vi "mobility_subvi_07_12a_JW.vi"(9 "NumPts":dbl=5.0, 11 "Path":path) -> (0 "Index-Lin":dbl, 1 "Index-Sat":dbl, 2 "Output":T1, 3 "XY Graph-Sat":cluster{dbl[], dbl[]}[](graph))   [LabVIEW 2011]
uses:
  <vilib>/Utility/file.llb/Read From Spreadsheet File (string).vi
  <vilib>/Analysis/NI_AALPro.lvlib
panel:
  out "XY Graph-Lin":cluster{dbl[], dbl[]}[](graph)
  out "ID Column 2":string[][](table)
  out "Capacitance (C)":dbl
  out "Numeric":dbl
  out "Dielectric (nm)":string
  out "Dielectric (d)":dbl
  out "Width":dbl
  out "Length":dbl
  out "ID Column 3":string[][](table)
  out "Vg Column":string[][](table)
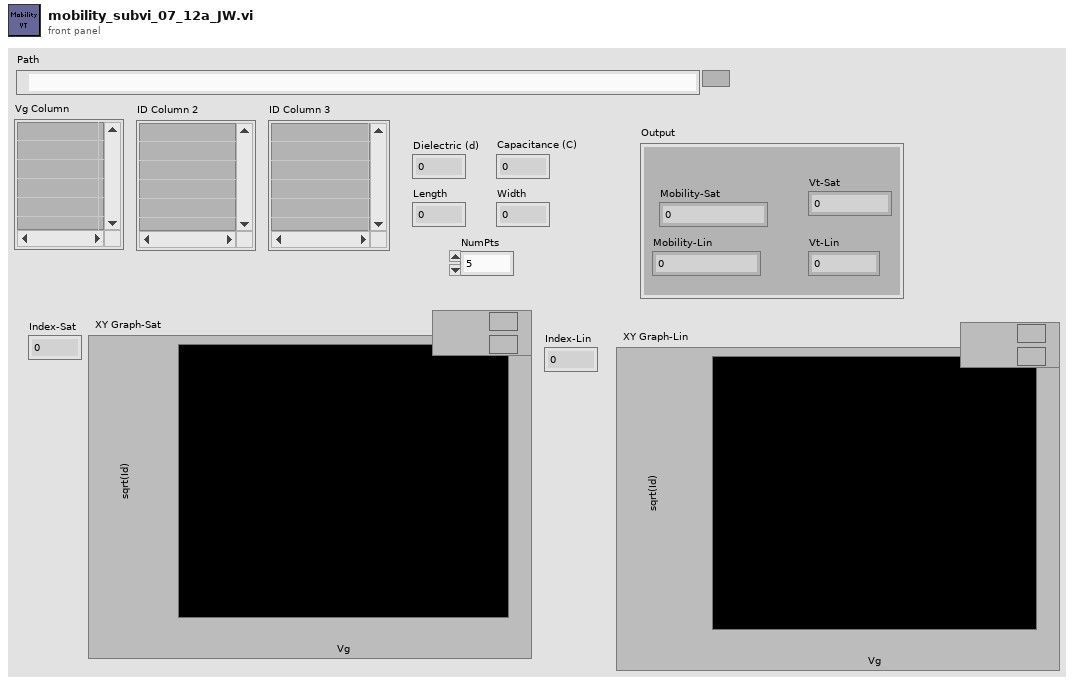
[diagram p1: front panel]
types:
  T1 = cluster{"Mobility-Sat":dbl, "Vt-Sat":dbl, "Vt-Lin":dbl, "Mobility-Lin":dbl}
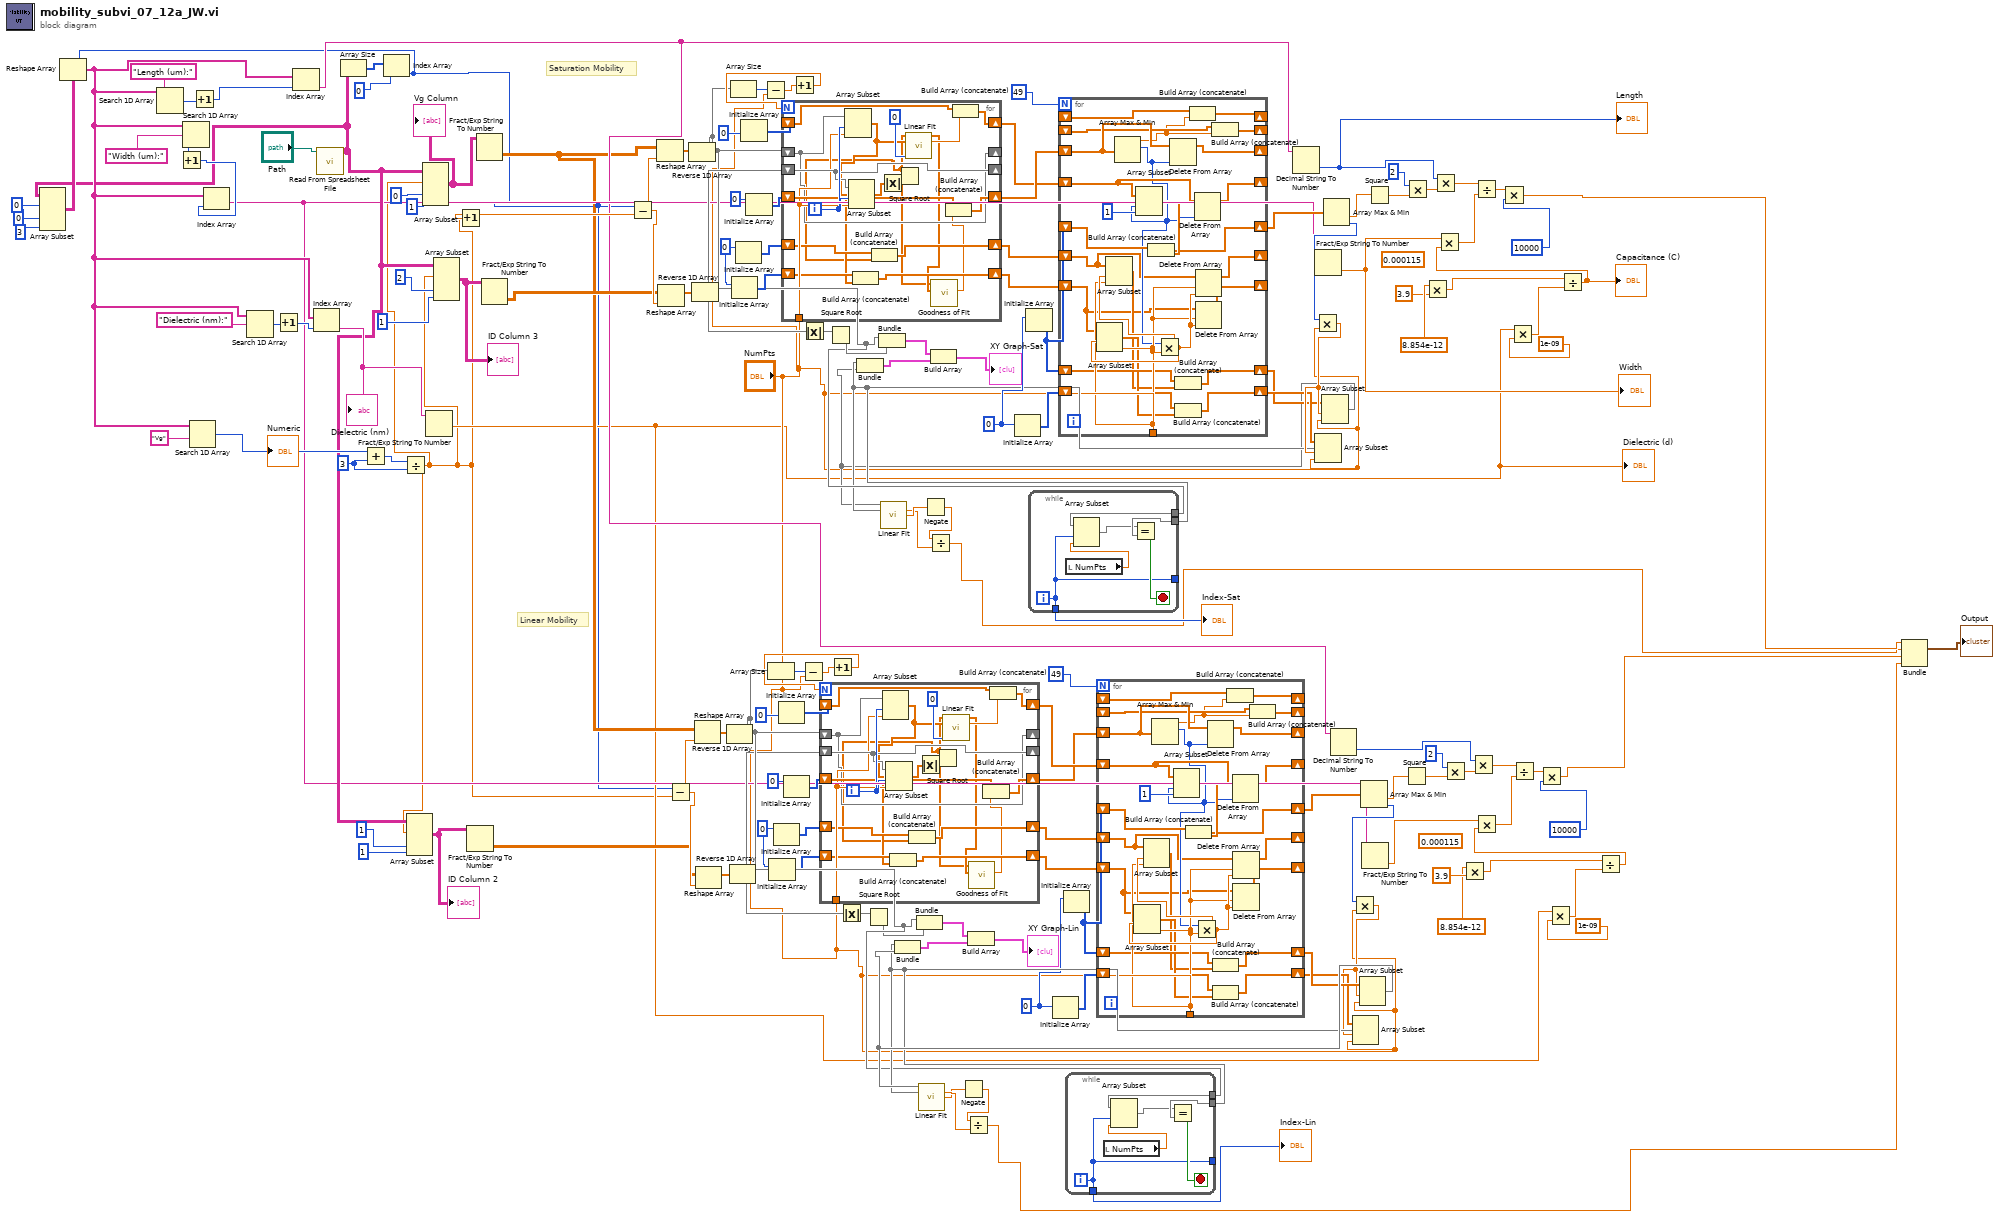
[diagram p0: block diagram]
diagram:
  w24 = 0
  w33 = 0
  (unwired) 0.000115
  w75 = 3
  w146 = 0
  w137 = 0
  (unwired) 0.000115
  # "Linear Mobility"
  # "Saturation Mobility"
  n1 = call-poly <vilib>:"Read From Spreadsheet File.vi"("file path (dialog if empty)"="Path") -> ("all rows"=w72:string[][])  [unwired: 6 in, 4 out]
  n2 = Array Subset(array=w72, index (row)=0, index (col)=0, length (col)=3) -> (w122:string[][])  [unwired: 1 in]
  n3 = Array Size(array=w72) -> (size(s)=w127:i32[])
  n4 = Index Array(array=w127, index=0) -> (element=w6:i32)
  n5 = Reshape Array(w122, w6) -> (w74:string[])
  n6 = Search 1D Array(1D array=w74, element="Length (um):") -> (index of element=w115:i32)  [unwired: 1 in]
  n7 = Search 1D Array(1D array=w74, element="Width (um):") -> (index of element=w116:i32)  [unwired: 1 in]
  n8 = Increment(x=w116) -> (x+1=w120:i32)
  n9 = Search 1D Array(1D array=w74, element="Vg") -> (index of element=w77:i32)  [unwired: 1 in]
  "Numeric" <- w77
  n10 = Increment(x=w115) -> (x+1=w118:i32)
  n11 = Index Array(array=w74, index=w120) -> (element=w13:string)
  n12 = Search 1D Array(1D array=w74, element="Dielectric (nm):") -> (index of element=w86:i32)  [unwired: 1 in]
  n13 = Increment(x=w86) -> (x+1=w85:i32)
  n14 = Index Array(array=w74, index=w118) -> (element=w12:string)
  n15 = Index Array(array=w74, index=w85) -> (element=w84:string)
  "Dielectric (nm)" <- w84
  n16 = Add(x=w77, y=w75) -> (x+y=w76:i32)
  n17 = Divide(x=w76, y=w75) -> (x/y=w7:dbl)
  n18 = Array Subset(array=w72, index (row)=w7, index (col)=1, length (col)=1) -> (w69:string[][])  [unwired: 1 in]
  "ID Column 2" <- w69
  n19 = Array Subset(array=w72, index (row)=w7, index (col)=0, length (col)=1) -> (w108:string[][])  [unwired: 1 in]
  "Vg Column" <- w108
  n20 = Fract/Exp String To Number(string=w84) -> (number=w8:dbl)  [unwired: 3 in, 1 out]
  "Dielectric (d)" <- w8
  n21 = Array Subset(array=w72, index (row)=w7, index (col)=2, length (col)=1) -> (w109:string[][])  [unwired: 1 in]
  "ID Column 3" <- w109
  n22 = Increment(x=w7) -> (x+1=w154:dbl)
  n23 = Fract/Exp String To Number(string=w69) -> (number=w9:dbl[][])  [unwired: 3 in, 1 out]
  n24 = Fract/Exp String To Number(string=w108) -> (number=w10:dbl[][])  [unwired: 3 in, 1 out]
  n25 = Fract/Exp String To Number(string=w109) -> (number=w110:dbl[][])  [unwired: 3 in, 1 out]
  n26 = Subtract(x=w6, y=w154) -> (x-y=w155:dbl)
  n27 = Reshape Array(w10, w155) -> (w142:dbl[])
  n28 = Reshape Array(w110, w155) -> (w143:dbl[])
  n29 = Subtract(x=w6, y=w7) -> (x-y=w16:dbl)
  n30 = Reverse 1D Array(array=w142) -> (reversed array=w89:dbl[])
  n31 = Reverse 1D Array(array=w143) -> (reversed array=w144:dbl[])
  n32 = Reshape Array(w10, w16) -> (w28:dbl[])
  n33 = Reshape Array(w9, w16) -> (w27:dbl[])
  n34 = Reverse 1D Array(array=w28) -> (reversed array=w61:dbl[])
  n35 = Reverse 1D Array(array=w27) -> (reversed array=w26:dbl[])
  n36 = Array Size(array=w89) -> (size(s)=w102:i32)
  n37 = Initialize Array(w137) -> (w139:i32[])  [unwired: 1 in]
  n38 = Initialize Array(w137) -> (w138:i32[])  [unwired: 1 in]
  n39 = Initialize Array(0) -> (w103:i32[])  [unwired: 1 in]
  n40 = Initialize Array(0) -> (w104:i32[])  [unwired: 1 in]
  n41 = Subtract(x=w102, y="NumPts") -> (x-y=w156:dbl)
  n42 = Array Size(array=w61) -> (size(s)=w53:i32)
  n43 = Initialize Array(w33) -> (w31:i32[])  [unwired: 1 in]
  n44 = Initialize Array(w33) -> (w32:i32[])  [unwired: 1 in]
  n45 = Initialize Array(0) -> (w52:i32[])  [unwired: 1 in]
  n46 = Initialize Array(0) -> (w51:i32[])  [unwired: 1 in]
  n47 = Increment(x=w156) -> (x+1=w157:dbl)
  n48 = for {
    N: w157 -> [_]
    shift-right: [w162] -> _
    shift-left: w89 -> [w162]
    shift-right: [w171] -> _
    shift-left: w144 -> [w171]
    shift-right: [w175] -> w112
    shift-left: w103 -> [w174]
    shift-right: [w173] -> w128
    shift-left: w104 -> [w172]
    tunnel: "NumPts" -> [w167]
    shift-right: [w165] -> w140
    shift-left: w138 -> [w166]
    shift-right: [w163] -> w141
    shift-left: w139 -> [w164]
    i -> [w177]
    n49 = Array Subset(array=w162, index=w177, length=w167) -> (w161:dbl[])
    n50 = Array Subset(array=w171, index=w177, length=w167) -> (w170:dbl[])
    n51 = Build Array (concatenate)(w164, w161) -> (w163:dbl[])
    n52 = Absolute Value(x=w170) -> (abs(x)=w169:dbl[])
    n53 = Square Root(x=w169) -> (sqrt(x)=w158:dbl[])
    n54 = Build Array (concatenate)(w166, w158) -> (w165:dbl[])
    n55 = call <vilib>:"Linear Fit.vi"("Y"=w158, "X"=w161, "method"=0) -> ("Best Linear Fit"=w160:dbl[], "slope"=w176:dbl)  [unwired: 8 in, 3 out]
    n56 = call <vilib>:"Goodness of Fit.vi"("Best Fit"=w160, "Y"=w158) -> ("R-square"=w159:dbl)  [unwired: 6 in, 3 out]
    n57 = Build Array (concatenate)(w172, w159) -> (w173:dbl[])
    n58 = Build Array (concatenate)(w174, w176) -> (w175:dbl[])
  }
  n59 = Subtract(x=w53, y="NumPts") -> (x-y=w15:dbl)
  n60 = Absolute Value(x=w144) -> (abs(x)=w136:dbl[])
  n61 = Square Root(x=w136) -> (sqrt(x)=w153:dbl[])
  n62 = Increment(x=w15) -> (x+1=w14:dbl)
  n63 = for {
    N: w14 -> [_]
    shift-right: [w182] -> _
    shift-left: w61 -> [w182]
    shift-right: [w191] -> _
    shift-left: w26 -> [w191]
    shift-right: [w195] -> w46
    shift-left: w52 -> [w194]
    shift-right: [w193] -> w42
    shift-left: w51 -> [w192]
    tunnel: "NumPts" -> [w187]
    shift-right: [w185] -> w30
    shift-left: w32 -> [w186]
    shift-right: [w183] -> w29
    shift-left: w31 -> [w184]
    i -> [w197]
    n64 = Array Subset(array=w182, index=w197, length=w187) -> (w181:dbl[])
    n65 = Array Subset(array=w191, index=w197, length=w187) -> (w190:dbl[])
    n66 = Build Array (concatenate)(w184, w181) -> (w183:dbl[])
    n67 = Absolute Value(x=w190) -> (abs(x)=w189:dbl[])
    n68 = Square Root(x=w189) -> (sqrt(x)=w178:dbl[])
    n69 = Build Array (concatenate)(w186, w178) -> (w185:dbl[])
    n70 = call <vilib>:"Linear Fit.vi"("Y"=w178, "X"=w181, "method"=0) -> ("Best Linear Fit"=w180:dbl[], "slope"=w196:dbl)  [unwired: 8 in, 3 out]
    n71 = call <vilib>:"Goodness of Fit.vi"("Best Fit"=w180, "Y"=w178) -> ("R-square"=w179:dbl)  [unwired: 6 in, 3 out]
    n72 = Build Array (concatenate)(w192, w179) -> (w193:dbl[])
    n73 = Build Array (concatenate)(w194, w196) -> (w195:dbl[])
  }
  n74 = Absolute Value(x=w26) -> (abs(x)=w34:dbl[])
  n75 = Square Root(x=w34) -> (sqrt(x)=w17:dbl[])
  n76 = Bundle(w89, w153) -> (w135:cluster{dbl[], dbl[]})  [unwired: 1 in]
  n77 = Bundle(w61, w17) -> (w35:cluster{dbl[], dbl[]})  [unwired: 1 in]
  n78 = Initialize Array(w146) -> (w145:i32[])  [unwired: 1 in]
  n79 = Initialize Array(w146) -> (w150:i32[])  [unwired: 1 in]
  n80 = Initialize Array(w24) -> (w25:i32[])  [unwired: 1 in]
  n81 = for {
    N: 49 -> [_]
    shift-right: [w222] -> _
    shift-left: w128 -> [w223]
    shift-right: [w202] -> _
    shift-left: w112 -> [w203]
    shift-right: [w219] -> w117
    shift-left: w150 -> [w218]
    shift-right: [w217] -> _
    shift-left: _ -> [w216]
    shift-right: [w215] -> _
    shift-left: _ -> [w214]
    shift-right: [w213] -> _
    shift-left: w140 -> [w199]
    shift-right: [w211] -> _
    shift-left: w141 -> [w198]
    tunnel: "NumPts" -> [w210]
    shift-right: [w209] -> w147
    shift-left: w150 -> [w208]
    shift-right: [w207] -> w148
    shift-left: w145 -> [w206]
    n82 = Array Max & Min(array=w223) -> (max value=w201:dbl, max index (indices)=w200:i32)  [unwired: 2 out]
    n83 = Array Subset(array=w203, index=w200, length=1) -> (w220:dbl[])
    n84 = Build Array (concatenate)(w218, w220) -> (w219:dbl[])
    n85 = Multiply(x=w200, y=w210) -> (x*y=w212:dbl)
    n86 = Array Subset(array=w198, index=w212, length=w210) -> (w205:dbl[])
    n87 = Array Subset(array=w199, index=w212, length=w210) -> (w204:dbl[])
    n88 = Delete From Array(array=w223, index=w200) -> (array with subset deleted=w222:dbl[])  [unwired: 1 in, 1 out]
    n89 = Build Array (concatenate)(w208, w204) -> (w209:dbl[])
    n90 = Build Array (concatenate)(w206, w205) -> (w207:dbl[])
    n91 = Build Array (concatenate)(w216, w201) -> (w217:dbl[])
    n92 = Delete From Array(array=w203, index=w200) -> (array with subset deleted=w202:dbl[])  [unwired: 1 in, 1 out]
    n93 = Delete From Array(array=w199, length=w210, index=w212) -> (array with subset deleted=w213:dbl[])  [unwired: 1 out]
    n94 = Delete From Array(array=w198, length=w210, index=w212) -> (array with subset deleted=w211:dbl[])  [unwired: 1 out]
    n95 = Build Array (concatenate)(w214, w201) -> (w215:dbl[])
  }
  n96 = Initialize Array(w24) -> (w20:i32[])  [unwired: 1 in]
  n97 = for {
    N: 49 -> [_]
    shift-right: [w248] -> _
    shift-left: w42 -> [w249]
    shift-right: [w228] -> _
    shift-left: w46 -> [w229]
    shift-right: [w245] -> w45
    shift-left: w20 -> [w244]
    shift-right: [w243] -> _
    shift-left: _ -> [w242]
    shift-right: [w241] -> _
    shift-left: _ -> [w240]
    shift-right: [w239] -> _
    shift-left: w30 -> [w225]
    shift-right: [w237] -> _
    shift-left: w29 -> [w224]
    tunnel: "NumPts" -> [w236]
    shift-right: [w235] -> w23
    shift-left: w20 -> [w234]
    shift-right: [w233] -> w22
    shift-left: w25 -> [w232]
    n98 = Array Max & Min(array=w249) -> (max value=w227:dbl, max index (indices)=w226:i32)  [unwired: 2 out]
    n99 = Array Subset(array=w229, index=w226, length=1) -> (w246:dbl[])
    n100 = Build Array (concatenate)(w244, w246) -> (w245:dbl[])
    n101 = Multiply(x=w226, y=w236) -> (x*y=w238:dbl)
    n102 = Array Subset(array=w224, index=w238, length=w236) -> (w231:dbl[])
    n103 = Array Subset(array=w225, index=w238, length=w236) -> (w230:dbl[])
    n104 = Delete From Array(array=w249, index=w226) -> (array with subset deleted=w248:dbl[])  [unwired: 1 in, 1 out]
    n105 = Build Array (concatenate)(w234, w230) -> (w235:dbl[])
    n106 = Build Array (concatenate)(w232, w231) -> (w233:dbl[])
    n107 = Build Array (concatenate)(w242, w227) -> (w243:dbl[])
    n108 = Delete From Array(array=w229, index=w226) -> (array with subset deleted=w228:dbl[])  [unwired: 1 in, 1 out]
    n109 = Delete From Array(array=w225, length=w236, index=w238) -> (array with subset deleted=w239:dbl[])  [unwired: 1 out]
    n110 = Delete From Array(array=w224, length=w236, index=w238) -> (array with subset deleted=w237:dbl[])  [unwired: 1 out]
    n111 = Build Array (concatenate)(w240, w227) -> (w241:dbl[])
  }
  n112 = Decimal String To Number(string=w12) -> (number=w119:i32)  [unwired: 2 in, 1 out]
  "Length" <- w119
  n113 = Fract/Exp String To Number(string=w13) -> (number=w121:dbl)  [unwired: 3 in, 1 out]
  "Width" <- w121
  n114 = Array Max & Min(array=w117) -> (min value=w107:dbl, min index (indices)=w149:i32)  [unwired: 2 out]
  n115 = Multiply(x=w149, y="NumPts") -> (x*y=w151:dbl)
  n116 = Array Subset(array=w148, index=w151, length="NumPts") -> (w83:dbl[])
  n117 = while {
    tunnel: [w250] -> _
    tunnel: w89 -> [w254]
    tunnel: w83 -> [w253]
    tunnel: [w250] -> w88
    i -> [w250]
    stop <- w255 stop-if-true
    n118 = local read "NumPts"() -> (w251:dbl)
    n119 = Array Subset(array=w254, index=w250, length=w251) -> (w252:dbl[])
    n120 = Equal?(x=w252, y=w253) -> (x = y?=w255:bool)
  }
  "Index-Sat" <- w88
  n121 = Array Subset(array=w147, index=w151, length="NumPts") -> (w82:dbl[])
  n122 = Bundle(w83, w82) -> (w152:cluster{dbl[], dbl[]})  [unwired: 1 in]
  n123 = call <vilib>:"Linear Fit.vi"("Y"=w82, "X"=w83) -> ("slope"=w79:dbl, "intercept"=w81:dbl)  [unwired: 9 in, 3 out]
  n124 = Negate(x=w81) -> (-x=w80:dbl)
  n125 = Divide(x=w80, y=w79) -> (x/y=w3:dbl)
  n126 = Build Array(w135, w152) -> (→"XY Graph-Sat":cluster{dbl[], dbl[]}[])
  n127 = Decimal String To Number(string=w12) -> (number=w44:i32)  [unwired: 2 in, 1 out]
  n128 = Array Max & Min(array=w45) -> (min value=w48:dbl, min index (indices)=w21:i32)  [unwired: 2 out]
  n129 = Multiply(x=w21, y="NumPts") -> (x*y=w19:dbl)
  n130 = Array Subset(array=w22, index=w19, length="NumPts") -> (w63:dbl[])
  n131 = while {
    tunnel: [w256] -> _
    tunnel: w61 -> [w260]
    tunnel: w63 -> [w259]
    tunnel: [w256] -> w62
    i -> [w256]
    stop <- w261 stop-if-true
    n132 = local read "NumPts"() -> (w257:dbl)
    n133 = Array Subset(array=w260, index=w256, length=w257) -> (w258:dbl[])
    n134 = Equal?(x=w258, y=w259) -> (x = y?=w261:bool)
  }
  "Index-Lin" <- w62
  n135 = Array Subset(array=w23, index=w19, length="NumPts") -> (w64:dbl[])
  n136 = Bundle(w63, w64) -> (w18:cluster{dbl[], dbl[]})  [unwired: 1 in]
  n137 = call <vilib>:"Linear Fit.vi"("Y"=w64, "X"=w63) -> ("slope"=w67:dbl, "intercept"=w65:dbl)  [unwired: 9 in, 3 out]
  n138 = Negate(x=w65) -> (-x=w66:dbl)
  n139 = Divide(x=w66, y=w67) -> (x/y=w1:dbl)
  n140 = Build Array(w35, w18) -> (→"XY Graph-Lin":cluster{dbl[], dbl[]}[])
  n141 = Fract/Exp String To Number(string=w13) -> (number=w43:dbl)  [unwired: 3 in, 1 out]
  n142 = Square(x=w107) -> (x^2=w101:dbl)
  n143 = Square(x=w48) -> (x^2=w54:dbl)
  n144 = Multiply(x=2, y=w101) -> (x*y=w100:dbl)
  n145 = Multiply(x=8.854e-12, y=3.9) -> (x*y=w133:dbl)
  n146 = Multiply(x=w119, y=w100) -> (x*y=w99:dbl)
  n147 = Multiply(x=2, y=w54) -> (x*y=w55:dbl)
  n148 = Multiply(x=8.854e-12, y=3.9) -> (x*y=w37:dbl)
  n149 = Multiply(x=w44, y=w55) -> (x*y=w56:dbl)
  n150 = Multiply(x=w8, y=1e-09) -> (x*y=w132:dbl)
  n151 = Multiply(x=w8, y=1e-09) -> (x*y=w38:dbl)
  n152 = Divide(x=w133, y=w132) -> (x/y=w73:dbl)
  "Capacitance (C)" <- w73
  n153 = Multiply(x=w121, y=w73) -> (x*y=w98:dbl)
  n154 = Divide(x=w99, y=w98) -> (x/y=w96:dbl)
  n155 = Multiply(x=w96, y=10000) -> (x*y=w4:dbl)
  n156 = Divide(x=w37, y=w38) -> (x/y=w68:dbl)
  n157 = Multiply(x=w43, y=w68) -> (x*y=w57:dbl)
  n158 = Divide(x=w56, y=w57) -> (x/y=w59:dbl)
  n159 = Multiply(x=w59, y=10000) -> (x*y=w2:dbl)
  n160 = Bundle(w4, w3, w2, w1) -> (→"Output":cluster{dbl, dbl, dbl, dbl})  [unwired: 1 in]
